vi "Get Element Labels by Regex.vi"(8 "error in":errorcluster, 9 "Exclude? (F)":bool, 10 "regular expression":string, 11 "Class in":refnum<class>) -> (0 "error out":errorcluster, 2 "Labels":string[](array[string]), 3 "Class out":refnum<class>)   [LabVIEW 2023, in "Label-Driven UI.lvlib"]
doc: "VI가 가진 모든 컨트롤과 인디케이터 중 정규표현식이 포함된 라벨들만 얻습니다.\nExclude?를 True로 설정할 경우, 입력된 정규표현식이 포함되지 않은 라벨들만 얻습니다."
uses:
  Label-Driven UI.lvlib
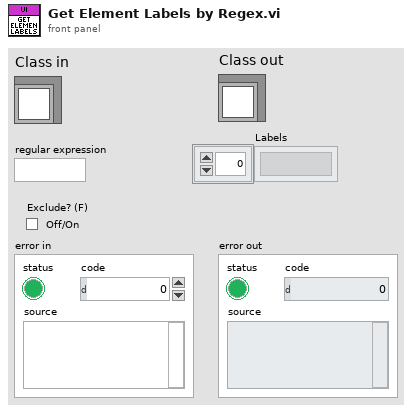
[diagram p1: front panel]
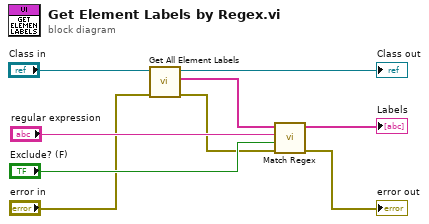
[diagram p0: block diagram]
diagram:
  n1 = call "Get All Element Labels.vi"("error in"="error in", "Class in"="Class in") -> ("error out"=w3:errorcluster, "Labels"=w7:string[], "Class out"=→"Class out":refnum<class>)  [unwired: 7 in]
  n2 = call "Match Regex.vi"("error in (no error)"=w3, "Exclude? (F)"="Exclude? (F)", "regular expression"="regular expression", "Labels"=w7) -> ("error out"=→"error out":errorcluster, "Array"=→"Labels":string[])  [unwired: 6 in]
